vi "bool to string small.vi"(7 "number":bool) -> (8 "String":string)   [LabVIEW 2018]
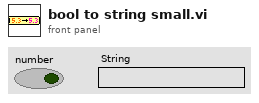
[diagram p1: front panel]
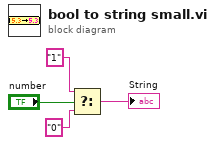
[diagram p0: block diagram]
diagram:
  n1 = Select(t="1" ("String"), s="number", f="0" ("String")) -> (s? t:f=→"String":string)
